vi "mqtt example gui.vi"() -> ()   [LabVIEW 2017]
uses:
  mqtt-LabVIEW/src/class/mqtt/mqttConfigFunction.ctl
  mqtt-LabVIEW/src/class/mqtt/mqtt.lvclass/mqtt.ctl
  mqtt-LabVIEW/src/class/mqtt/mqttTypedef/mqttSubscribeCluster.ctl
  mqtt-LabVIEW/src/class/mqtt/mqttTypedef/mqttQOSlevel.ctl
  mqtt payload to double.vi
  mqtt payload to boolean.vi
  mqtt-LabVIEW/src/class/mqtt/mqtt.lvclass
panel:
  in  "send client time":bool
  in  "auto reconnect":bool
  out "MQTT Subscribed":bool
  out "MQTT Connection":bool
  out "RX Topic":string
  out "RX Value":string
  in  "boolean control":bool
  out "boolean indicator":bool
  out "numeric indicator":dbl min=24.6 max=310.0 format="%0.3f"
  in  "send instruction":bool
  in  "numeric control":dbl format="%0.3f"
  out "messageID":u16
  out "quit":bool
  # "MQTT related"
  # "Last received message"
  # "Example program functions"
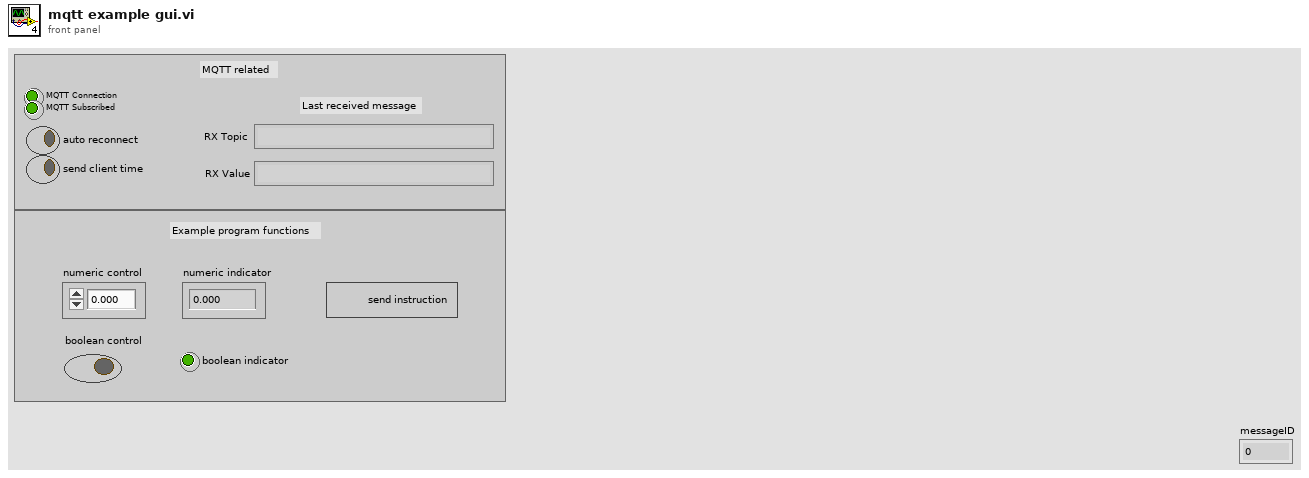
[diagram p1: front panel]
types:
  T1 = enum8{"Enabled", "Disabled", "Disabled and Grayed Out"}
  T2 = typedef "mqtt.lvclass/mqttConfigFunction.ctl" = enum16{"init", "deinit", "set", "get"}
  T3 = typedef "mqttSubscribeCluster.ctl" = cluster{"Topic":string, "QoS":T4}
  T4 = typedef "mqttQOSlevel.ctl" = enum8{"At most once", "At least once", "Exactly once", "Reserved"}
  T5 = typedef "mqttUserInformation.ctl" = cluster{"Will message":string, "Will Topic":string}
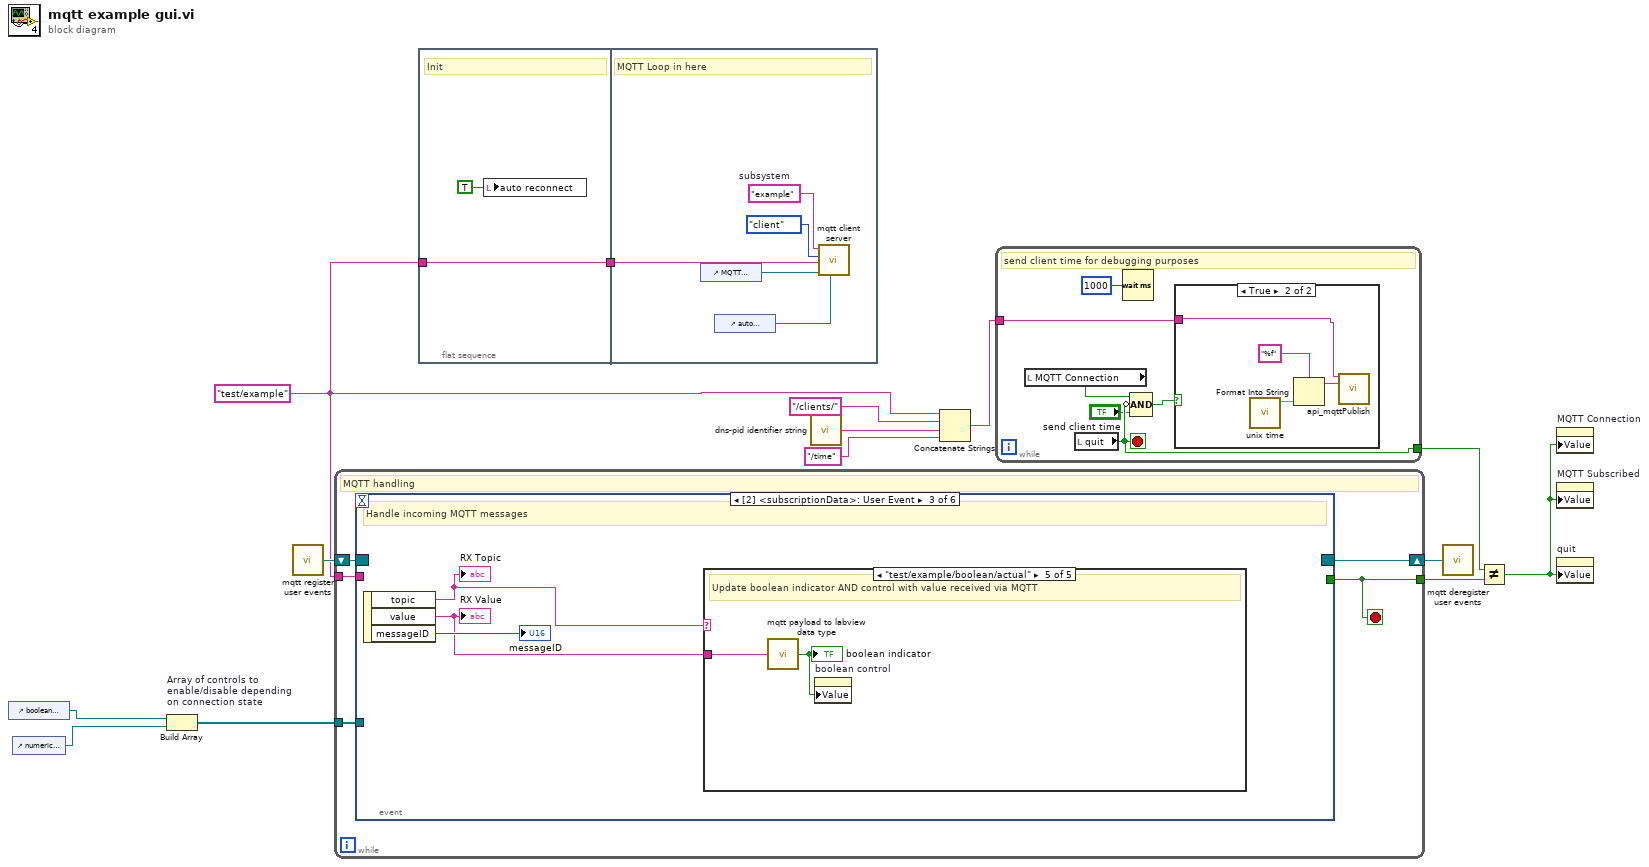
[diagram p0: block diagram]
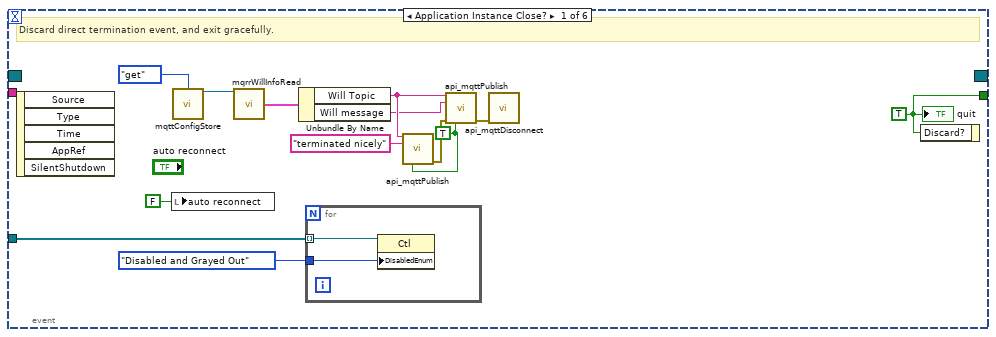
[diagram p3: hidden frame]
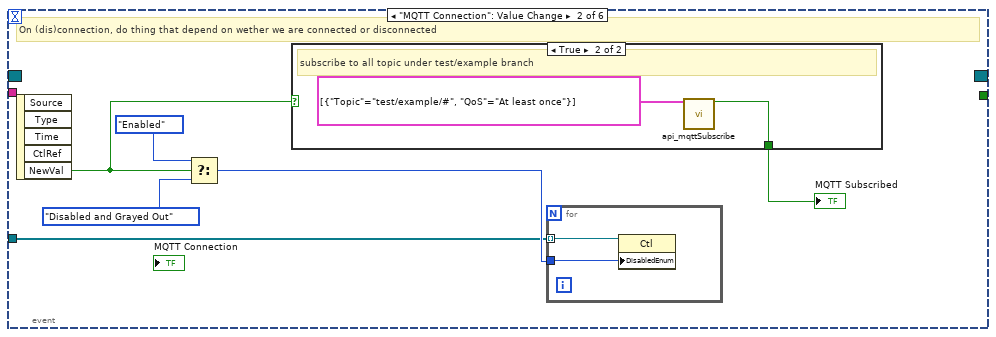
[diagram p4: hidden frame]
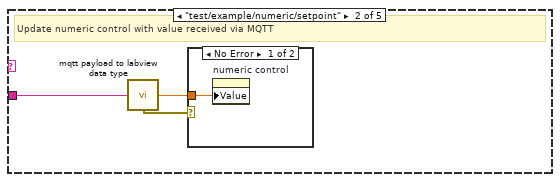
[diagram p7: hidden frame]
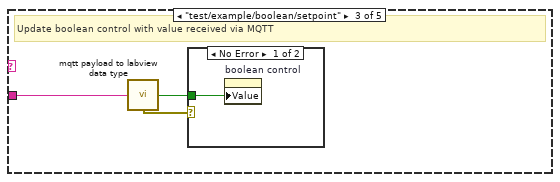
[diagram p9: hidden frame]
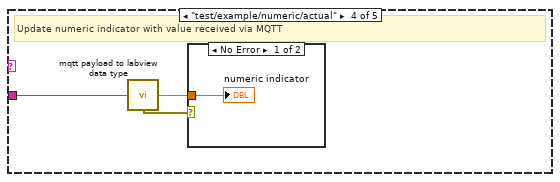
[diagram p11: hidden frame]
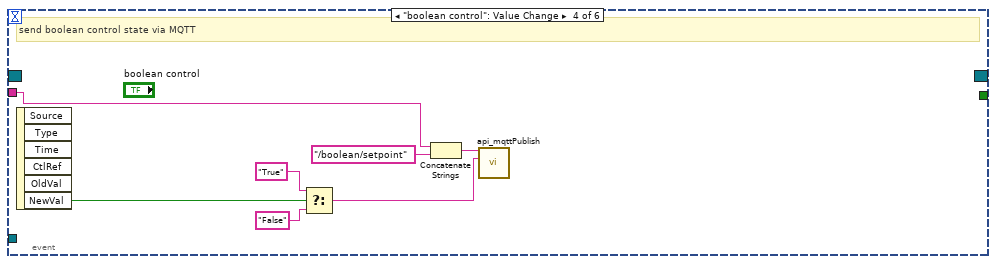
[diagram p13: hidden frame]
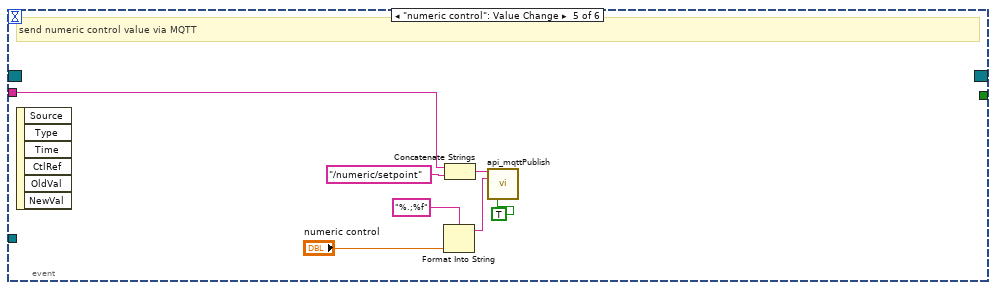
[diagram p14: hidden frame]
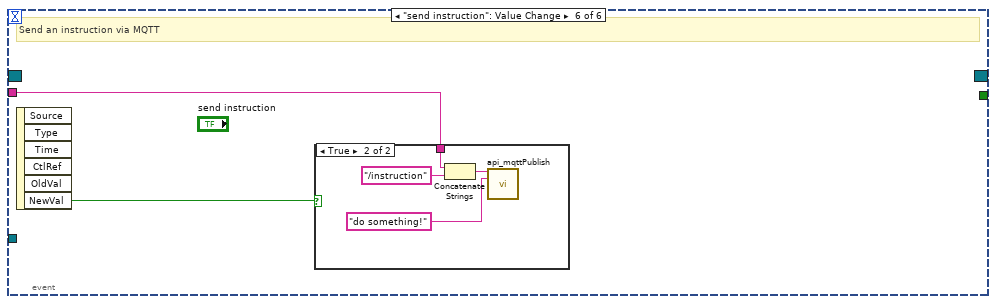
[diagram p15: hidden frame]
diagram:
  w1 = "test/example" ("mqtt prefix")
  n1 = control-ref of="boolean control"() -> (w3:refnum<vi>)
  n2 = control-ref of="numeric control"() -> (w5:refnum<vi>)
  n3 = Build Array "Array of controls to \nenable/disable depending \non connection state"(w3, w5) -> (w4:refnum<vi>[])
  n4 = call "mqtt register user events.vi"() -> ("Event Registration Refnum"=w14:refnum<event-registration>)  [unwired: 1 in]
  n5 = while {
    shift-right: [w18] -> w13
    shift-left: w14 -> [w19]
    tunnel: [w17] -> w12
    tunnel: w4 -> [w16]
    tunnel: w1 -> [w15]
    stop <- w17 stop-if-true
    # "MQTT handling"
    n6 = event shown="[2] <subscriptionData>: User Event" {
      selector: w19 -> [_ _ _ _ _ _]
      dyn-events: [_ _ _ _ _ _] -> w18
      timeout: _ -> [_ _ _ _ _ _]
      tunnel: [w20 _ _ _ _ _] -> w17
      tunnel: w15 -> [_ _ _ w63 w76 w78]
      tunnel: w16 -> [w23 w37 _ _ _ _]
      event Application Instance Close? {
        w20 = TRUE ("quit")
        w24 = TRUE ("retain(F)")
        # "Discard direct termination event, and exit gracefully."
        n7 = event-data() -> ()  [unwired: 1 in, 5 out]
        n8 = local write "auto reconnect"(FALSE ("keep connected")) -> ()
        n9 = call "mqttConfigStore.vi"("function"=mqttConfigFunction."get") -> ("mqtt.lvclass out"=w30:refnum<class "mqtt.lvclass">)  [unwired: 13 in, 1 out]
        n10 = call "mqrrWillInfoRead.vi"("mqtt in"=w30) -> ("Will Info"=w32:T5)  [unwired: 12 in, 2 out]
        n11 = Unbundle By Name(w32) -> ("Will Topic"=w26:string, "Will message"=w25:string)
        n12 = for {
          tunnel: w23 -> [w34] mode=indexing
          tunnel: T1."Disabled and Grayed Out" ("Disabled") -> [w33]
          n13 = property class="Ctl"(reference=w34, "DisabledEnum"=w33) -> ()  [unwired: 1 in, 2 out]
        }
        n14 = call "api_mqttPublish.vi"("topic"=w26, "value"="terminated nicely", "retain(F)"=w24) -> ("error out"=w28:errorcluster)  [unwired: 11 in, 1 out]
        n15 = call "api_mqttPublish.vi"("topic"=w26, "value"=w25, "error in (no error)"=w28, "retain(F)"=w24) -> ("error out"=w27:errorcluster)  [unwired: 10 in, 1 out]
        n16 = call "api_mqttDisconnect.vi"("error in (no error)"=w27) -> ()  [unwired: 13 in, 2 out]
        n17 = event-data("Discard?"=w20) -> ()  [unwired: 1 in, 1 out]
        "quit" <- w20
      }
      event "MQTT Connection": Value Change {
        # "On (dis)connection, do thing that depend on wether we are connected or disconnected"
        n18 = event-data() -> ("NewVal"=w36:bool)  [unwired: 1 in, 4 out]
        n19 = Select(t=T1."Enabled" ("Disabled"), s=w36, f=T1."Disabled and Grayed Out") -> (s? t:f=w38:T1)
        n20 = case shown="True" w36 {
          selector: w36 -> [w41 _]
          tunnel: [w41 w42] -> w35
          frame False {
          }
          frame True {
            # "subscribe to all topic under test/example branch"
            n21 = call "api_mqttSubscribe.vi"("subscriptionInfo"=T3[] [{"Topic"="test/example/#", "QoS"=enum."At least once"}] ("subscriptionInfo 2")) -> ("success"=w42:bool)  [unwired: 13 in, 1 out]
          }
        }
        "MQTT Subscribed" <- w35
        n22 = for {
          tunnel: w37 -> [w45] mode=indexing
          tunnel: w38 -> [w44]
          n23 = property class="Ctl"(reference=w45, "DisabledEnum"=w44) -> ()  [unwired: 1 in, 2 out]
        }
      }
      event User Event {
        # "Handle incoming MQTT messages"
        n24 = event-data() -> ("topic"=w47:string, "value"=w46:string, "messageID"=→"messageID":u16)  [unwired: 1 in]
        "RX Topic" <- w47
        "RX Value" <- w46
        n25 = case shown="\"test/example/boolean/actual\"" w47 {
          tunnel: w46 -> [_ w51 w55 w59 w62]
          frame Default {
          }
          frame "test/example/numeric/setpoint" {
            # "Update numeric control with value received via MQTT"
            n26 = call-poly "mqtt payload to labview data type.vi"("MQTT payload"=w51) -> ("double"=w50:dbl, "error out"=w49:errorcluster)  [unwired: 13 in]
            n27 = case shown="No Error" w49 {
              tunnel: w50 -> [w52 _]
              frame No Error {
                n28 = property on="numeric control" class="DigNum (strict)"("Value"=w52) -> ()  [unwired: 2 in, 2 out]
              }
              frame Error {
              }
            }
          }
          frame "test/example/boolean/setpoint" {
            # "Update boolean control with value received via MQTT"
            n29 = call-poly "mqtt payload to labview data type.vi"("String"=w55) -> ("Boolean"=w54:bool, "error out"=w53:errorcluster)  [unwired: 13 in]
            n30 = case shown="No Error" w53 {
              tunnel: w54 -> [w56 _]
              frame No Error {
                n31 = property on="boolean control" class="Bool (strict)"("Value"=w56) -> ()  [unwired: 2 in, 2 out]
              }
              frame Error {
              }
            }
          }
          frame "test/example/numeric/actual" {
            # "Update numeric indicator with value received via MQTT"
            n32 = call-poly "mqtt payload to labview data type.vi"("MQTT payload"=w59) -> ("double"=w58:dbl, "error out"=w57:errorcluster)  [unwired: 13 in]
            n33 = case shown="No Error" w57 {
              tunnel: w58 -> [w60 _]
              frame No Error {
                "numeric indicator" <- w60
              }
              frame Error {
              }
            }
          }
          frame "test/example/boolean/actual" {
            # "Update boolean indicator AND control with value received via MQTT"
            n34 = call-poly "mqtt payload to labview data type.vi"("String"=w62) -> ("Boolean"=w61:bool)  [unwired: 13 in, 1 out]
            "boolean indicator" <- w61
            n35 = property on="boolean control" class="Bool (strict)"("Value"=w61) -> ()  [unwired: 2 in, 2 out]
          }
        }
      }
      event "boolean control": Value Change {
        # "send boolean control state via MQTT"
        n36 = event-data() -> ("NewVal"=w67:bool)  [unwired: 1 in, 5 out]
        n37 = Select(t="True" ("string"), s=w67, f="False" ("string")) -> (s? t:f=w64:string)
        n38 = Concatenate Strings(w63, "/boolean/setpoint" ("string")) -> (w69:string)
        n39 = call "api_mqttPublish.vi"("topic"=w69, "value"=w64) -> ()  [unwired: 12 in, 2 out]
      }
      event "numeric control": Value Change {
        # "send numeric control value via MQTT"
        n40 = event-data() -> ()  [unwired: 1 in, 6 out]
        n41 = Format Into String(format string="%.;%f", "numeric control") -> (resulting string=w73:string)  [unwired: 2 in, 1 out]
        n42 = Concatenate Strings(w76, "/numeric/setpoint" ("string")) -> (w75:string)
        n43 = call "api_mqttPublish.vi"("topic"=w75, "value"=w73, "retain(F)"=TRUE) -> ()  [unwired: 11 in, 2 out]
      }
      event "send instruction": Value Change {
        # "Send an instruction via MQTT"
        n44 = event-data() -> ("NewVal"=w77:bool)  [unwired: 1 in, 5 out]
        n45 = case shown="True" w77 {
          tunnel: w78 -> [_ w82]
          frame False {
          }
          frame True {
            n46 = Concatenate Strings(w82, "/instruction" ("string")) -> (w81:string)
            n47 = call "api_mqttPublish.vi"("topic"=w81, "value"="do something!" ("string")) -> ()  [unwired: 12 in, 2 out]
          }
        }
      }
    }
  }
  n48 = flat-sequence {
    tunnel: [w83] -> w2
    tunnel: w1 -> [w83]
    tunnel: w2 -> [w87]
    frame #0 {
      # "Init"
      n49 = local write "auto reconnect"(TRUE ("keep connected")) -> ()
    }
    frame #1 {
      w85 = "example"  # subsystem
      # "MQTT Loop in here"
      n50 = control-ref of="MQTT Connection"() -> (w88:refnum<vi>)
      n51 = control-ref of="auto reconnect"() -> (w89:refnum<vi>)
      n52 = call "mqtt client server.vi"("keep connected"=w89, "connect success reference"=w88, "mqtt prefix"=w87, "client or server"=enum16{"client", "server"}."client", "subsystem"=w85) -> ()  [unwired: 6 in, 1 out]
    }
  }
  n53 = call "dns-pid identifier string.vi"() -> ("DNS_PID Identifier string"=w9:string)  [unwired: 1 in]
  n54 = Concatenate Strings(w1, "/clients/" ("string"), w9, "/time" ("string")) -> (w7:string)
  n55 = while {
    tunnel: [w93] -> w11
    tunnel: w7 -> [w91]
    stop <- w93 stop-if-true
    # "send client time for debugging purposes"
    n56 = local read "MQTT Connection"() -> (w94:bool)
    n57 = local read "quit"() -> (w93:bool)
    n58 = Wait (ms)(milliseconds to wait=u32 1000) -> ()  [unwired: 1 out]
    n59 = Compound Arithmetic op=AND(w94, invert w93, "send client time") -> (w92:bool)
    n60 = case shown="True" w92 {
      tunnel: w91 -> [_ w96]
      frame False {
      }
      frame True {
        n61 = call "unix time.vi"() -> ("Unix time"=w98:dbl)  [unwired: 10 in, 1 out]
        n62 = Format Into String(format string="%f", w98) -> (resulting string=w97:string)  [unwired: 2 in, 1 out]
        n63 = call "api_mqttPublish.vi"("topic"=w96, "value"=w97) -> ()  [unwired: 12 in, 2 out]
      }
    }
  }
  n64 = call "mqtt deregister user events.vi"("Event Registration Refnum in"=w13) -> ()  [unwired: 1 in]
  n65 = Not Equal?(x=w11, y=w12) -> (x != y?=w6:bool)
  n66 = property on="MQTT Connection" class="Bool (strict)"("Value"=w6) -> ()  [unwired: 2 in, 2 out]
  n67 = property on="MQTT Subscribed" class="Bool (strict)"("Value"=w6) -> ()  [unwired: 2 in, 2 out]
  n68 = property on="quit" class="Bool (strict)"("Value"=w6) -> ()  [unwired: 2 in, 2 out]
